vi "ask.vi"(0 "agent_simple_qa in":refnum<class "agent_simple_qa.lvclass">, 5 "message_text":refnum<class "message_text.lvclass">, 11 "error in (no error)":errorcluster) -> (4 "agent_simple_qa out":refnum<class "agent_simple_qa.lvclass">, 6 "message_text_response":refnum<class "message_text.lvclass">, 15 "error out":errorcluster)   [LabVIEW 2020, in "agent_simple_qa.lvclass"]
uses:
  agent_simple_qa.lvclass
  models/message_text/message_text.lvclass
  D:/petwork/labview-llm-libraries/src/models/abstract_message_base/abstract_message_base.lvclass
  agent_simple_qa.lvclass/agent_simple_qa.ctl
  models/message_vectors/message_vectors.lvclass
  models/message_vectors/get_vector_message_value.vi
  vectorstore/abstract_vector_base/abstract_vector_base.lvclass
  models/abstract_llm_chatcompletion/abstract_llm_chatcompletion.lvclass
  models/abstract_llm_embedding/abstract_llm_embedding.lvclass
  D:/petwork/labview-llm-libraries/src/models/message_vectors/message_vectors.lvclass
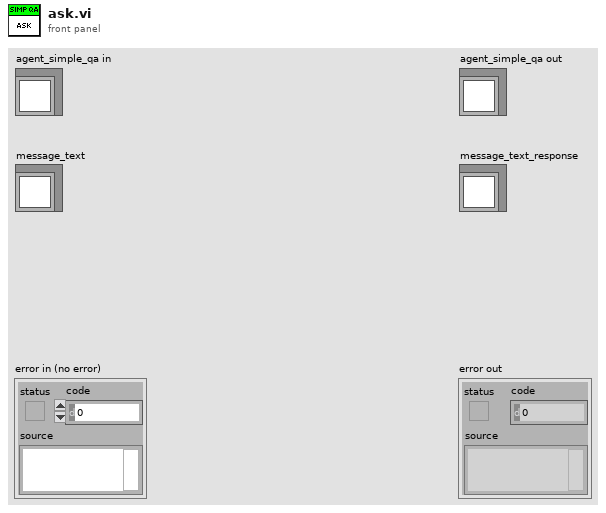
[diagram p1: front panel]
types:
  T1 = typedef "message_vectors.lvclass/embedding.ctl" = cluster{"index":u32, "Vectors":dbl[]}
  T2 = typedef "abstract_vector_base.lvclass/search result.ctl" = cluster{"score":dbl, "vector":T3}
  T3 = typedef "abstract_vector_base.lvclass/vector.ctl" = cluster{"id":string, "vector":dbl[], "text":string, "metadata":cluster{"key":string, "value":string}[]}
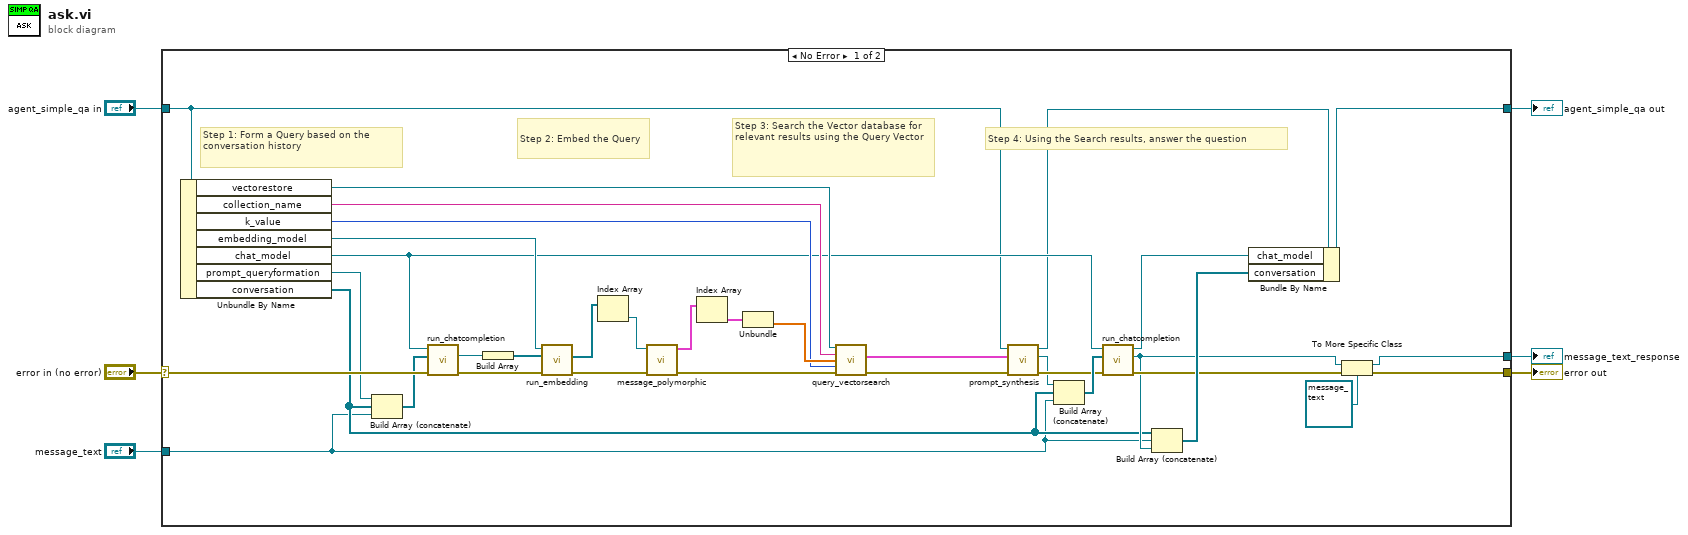
[diagram p0: block diagram]
diagram:
  n1 = case shown="No Error" "error in (no error)" {
    selector: "error in (no error)" -> [w32 w43]
    tunnel: [w36 w43] -> w5
    tunnel: [w40 w42] -> w3
    tunnel: "agent_simple_qa in" -> [w12 w42]
    tunnel: "message_text" -> [w7 _]
    tunnel: [w33 _] -> w1
    frame No Error {
      # "Step 4: Using the Search results, answer the question"
      # "Step 2: Embed the Query"
      # "Step 3: Search the Vector database for relevant results using the Query Vector"
      # "Step 1: Form a Query based on the conversation history"
      n2 = Unbundle By Name(w12) -> ("vectorestore"=w29:refnum<class "abstract_vector_base.lvclass">, "collection_name"=w28:string, "k_value"=w16:u32, "embedding_model"=w27:refnum<class "abstract_llm_base.lvclass">, "chat_model"=w15:refnum<class "abstract_llm_base.lvclass">, "prompt_queryformation"=w30:refnum<class "message_text.lvclass">, "conversation"=w8:refnum<class "abstract_message_base.lvclass">[])
      n3 = Build Array (concatenate)(w30, w8, w7) -> (w31:refnum<class "abstract_message_base.lvclass">[])
      n4 = call "run_chatcompletion.vi"("error in (no error)"=w32, "Messages"=w31, "abstract_llm_chatcompletion in"=w15) -> ("error out"=w26:errorcluster, "Response"=w25:refnum<class "abstract_message_base.lvclass">)  [unwired: 6 in, 1 out]
      n5 = Build Array(w25) -> (w24:refnum<class "abstract_message_base.lvclass">[])
      n6 = call "run_embedding.vi"("error in (no error)"=w26, "Messages"=w24, "abstract_llm_embedding in"=w27) -> ("error out"=w21:errorcluster, "Response"=w23:refnum<class "message_vectors.lvclass">[])  [unwired: 6 in, 1 out]
      n7 = Index Array(array=w23) -> (element=w22:refnum<class "message_vectors.lvclass">)  [unwired: 1 in]
      n8 = call-poly "message_polymorphic.vi"("error in (no error)"=w21, "message_vectors in"=w22) -> ("error out"=w17:errorcluster, "embedding_data"=w20:T1[])  [unwired: 8 in]
      n9 = Index Array(array=w20) -> (element=w19:T1)  [unwired: 1 in]
      n10 = Unbundle(w19) -> ("Vectors"=w18:dbl[])  [unwired: 1 out]
      n11 = call-dynamic "query_vectorsearch.vi"("abstract_vector_base in"=w29, "collection_name"=w28, "vector"=w18, "limit"=w16, "error in (no error)"=w17) -> ("results"=w10:T2[], "error out"=w14:errorcluster)  [unwired: 8 in, 1 out]
      n12 = call "prompt_synthesis.vi"("error in (no error)"=w14, "search_results"=w10, "agent_simple_qa in"=w12) -> ("error out"=w13:errorcluster, "prompt_synthesiser"=w9:refnum<class "message_text.lvclass">, "agent_simple_qa out"=w11:refnum<class "agent_simple_qa.lvclass">)  [unwired: 6 in]
      n13 = Build Array (concatenate)(w9, w8, w7) -> (w39:refnum<class "abstract_message_base.lvclass">[])
      n14 = call "run_chatcompletion.vi"("error in (no error)"=w13, "Messages"=w39, "abstract_llm_chatcompletion in"=w15) -> ("error out"=w37:errorcluster, "Response"=w35:refnum<class "abstract_message_base.lvclass">, "abstract_llm_chatcompletion out"=w41:refnum<class "abstract_llm_base.lvclass">)  [unwired: 6 in]
      n15 = Build Array (concatenate)(w8, w7, w35) -> (w38:refnum<class "abstract_message_base.lvclass">[])
      n16 = Bundle By Name(cluster=w11, "chat_model"=w41, "conversation"=w38) -> (w40:refnum<class "agent_simple_qa.lvclass">)
      n17 = To More Specific Class(target class=refnum<class "message_text.lvclass"> refnum ("message_text"), reference=w35, error in=w37) -> (specific class reference=w33:refnum<class "message_text.lvclass">, error out=w36:errorcluster)
    }
    frame Error {
    }
  }
  "error out" <- w5
  "agent_simple_qa out" <- w3
  "message_text_response" <- w1
